vi "lv-getBuildSpec.vi"(8 "error in (no error)":errorcluster, 9 "Build specification":string="Package", 10 "Target":string="My Computer", 11 "LabVIEW Project Path":path=path "C:/Users/admin/Desktop/Source/Waveform-Processing-Custom-Device.lvproj") -> (0 "error out":errorcluster={"status"=TRUE, "code"=1055, "source"="Property Node in lv-cli-steps.lvlib:lv-getBuildSpec.vi"}, 3 "Project refs":T1={"LabVIEW Project Path"=path "C:/Users/admin/Desktop/Source/Waveform-Processing-Custom-Device.lvproj", "Project refnum"=refnum, "Build spec refnum"=refnum})   [LabVIEW 2014, in "veristand-steps-build-system.lvlib"]
uses:
  veristand-steps-build-system.lvlib
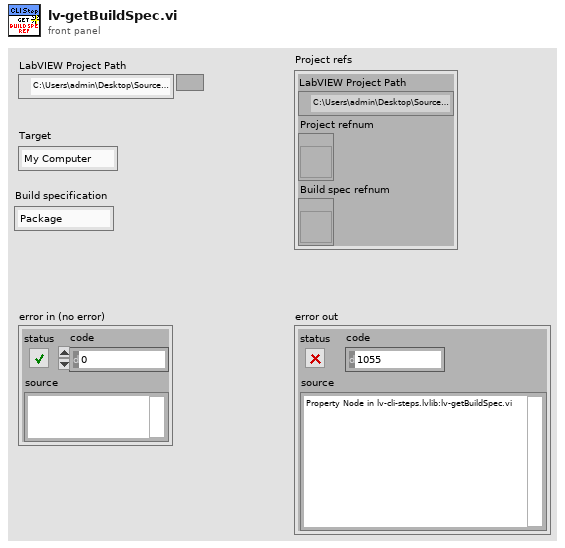
[diagram p1: front panel]
types:
  T1 = cluster{"LabVIEW Project Path":path, "Project refnum":refnum<vi>, "Build spec refnum":refnum<vi>}
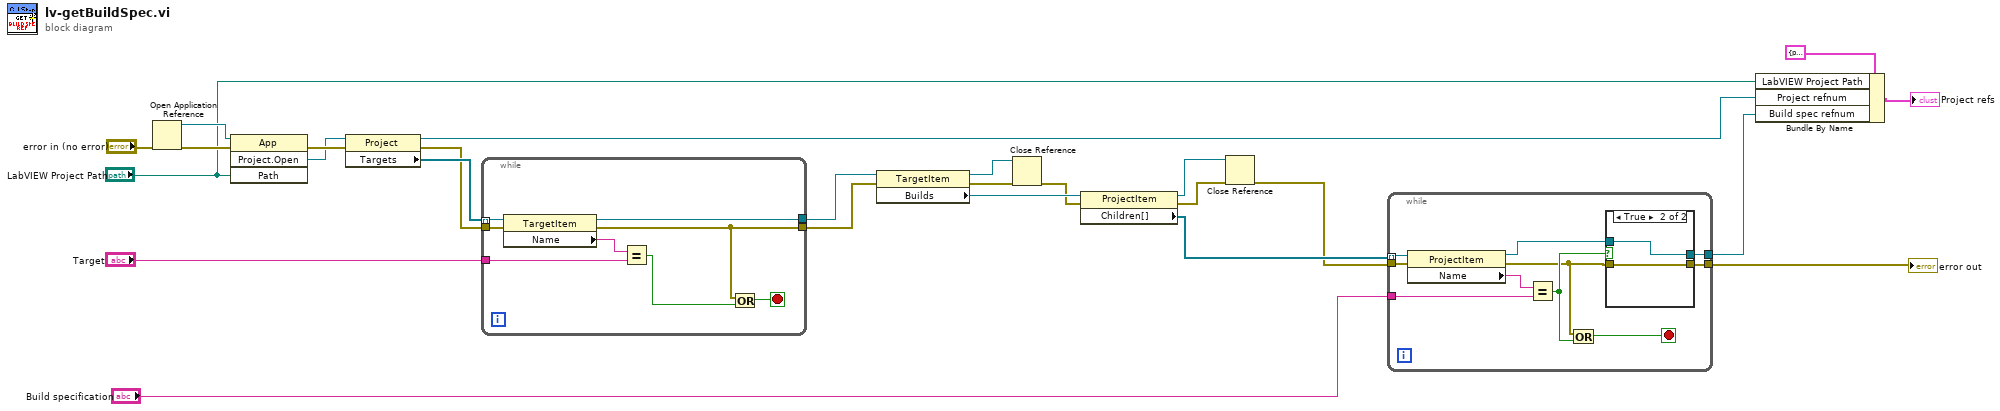
[diagram p0: block diagram]
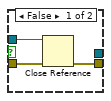
[diagram p2: hidden frame]
diagram:
  n1 = Open Application Reference(8:"error in (no error)") -> (0:w25:errorcluster, 3:w24:refnum<vi>)  [unwired: 3 in]
  n2 = invoke class="App" method="Project.Open"(reference=w24, error in=w25, "Path"="LabVIEW Project Path") -> (error out=w23:errorcluster, "Project:Open"=w22:refnum<vi>)  [unwired: 1 in, 2 out]
  n3 = property class="Project"(reference=w22, error in=w23) -> (reference out=w3:refnum<vi>, error out=w12:errorcluster, "Targets"=w14:refnum<vi>[])
  n4 = while {
    tunnel: w14 -> [w33] mode=indexing
    tunnel: "Target" -> [w31]
    tunnel: [w29] -> w11
    tunnel: w12 -> [w28]
    tunnel: [w27] -> w10
    stop <- w26 stop-if-true
    n5 = property class="TargetItem"(reference=w33, error in=w28) -> (reference out=w27:refnum<vi>, error out=w29:errorcluster, "Name"=w32:string)
    n6 = Equal?(x=w32, y=w31) -> (x = y?=w30:bool)
    n7 = Or(x=w29, y=w30) -> (x .or. y?=w26:bool)
  }
  n8 = property class="TargetItem"(reference=w10, error in=w11) -> (reference out=w19:refnum<vi>, error out=w20:errorcluster, "Builds"=w21:refnum<vi>)
  n9 = Close Reference(reference=w19, error in (no error)=w20) -> (error out=w18:errorcluster)
  n10 = property class="ProjectItem"(reference=w21, error in=w18) -> (reference out=w17:refnum<vi>, error out=w16:errorcluster, "Children[]"=w8:refnum<vi>[])
  n11 = Close Reference(reference=w17, error in (no error)=w16) -> (error out=w6:errorcluster)
  n12 = while {
    tunnel: w8 -> [w43] mode=indexing
    tunnel: "Build specification" -> [w41]
    tunnel: w6 -> [w40]
    tunnel: [w34] -> w2
    tunnel: [w35] -> w7
    stop <- w39 stop-if-true
    n13 = property class="ProjectItem"(reference=w43, error in=w40) -> (reference out=w36:refnum<vi>, error out=w37:errorcluster, "Name"=w42:string)
    n14 = Equal?(x=w42, y=w41) -> (x = y?=w38:bool)
    n15 = Or(x=w37, y=w38) -> (x .or. y?=w39:bool)
    n16 = case shown="True" w38 {
      tunnel: w37 -> [w46 w47]
      tunnel: w36 -> [w45 w48]
      tunnel: [w44 w47] -> w35
      tunnel: [_ w48] -> w34
      frame False {
        n17 = Close Reference(reference=w45, error in (no error)=w46) -> (error out=w44:errorcluster)
      }
      frame True {
      }
    }
  }
  "error out" <- w7
  n18 = Bundle By Name(cluster=T1 {"LabVIEW Project Path"=path "C:/Users/admin/Desktop/Source/Waveform-Processing-Custom-Device.lvproj", "Project refnum"=refnum, "Build spec refnum"=refnum} ("Project refs"), "LabVIEW Project Path"="LabVIEW Project Path", "Project refnum"=w3, "Build spec refnum"=w2) -> (→"Project refs":T1)
